vi "Relay.vi"(6 "Relay Mode":bool[](array[boolean]), 8 "error in":errorcluster, 9 "Relay Class":string="NI 6514\\NI 6514.lvclass", 10 "Line(s)":string="PXIe-6514/port4/line0:2", 11 "Base Path":path=path "C:/GitHub/OOP Template/HAL/Concrete") -> (0 "error out":errorcluster={"status"=TRUE, "code"=1446, "source"="Preserve Run-Time Class in MAL.lvlib:Relay.vi"})   [LabVIEW 2019, in "MAL.lvlib"]
uses:
  MAL.lvlib
  Hardware Abstraction/Harware Abstraction/DIO/DIO.lvclass
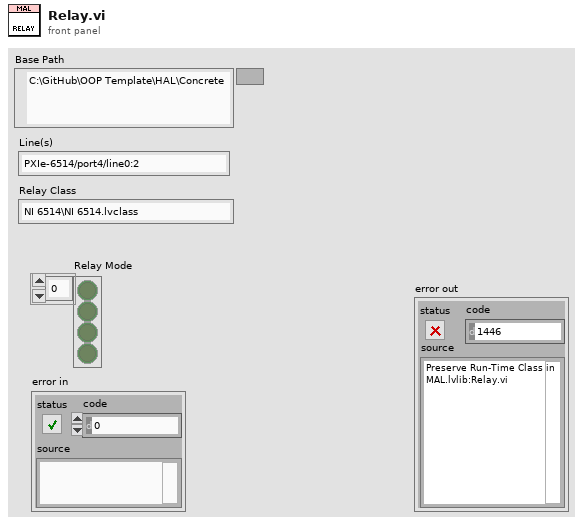
[diagram p1: front panel]
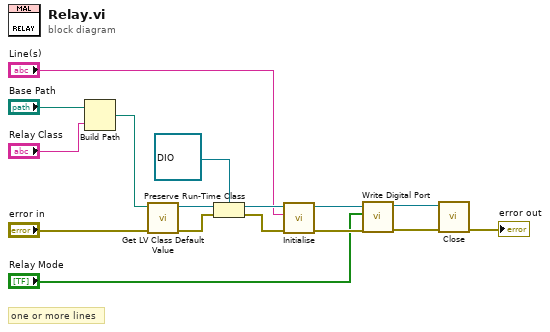
[diagram p0: block diagram]
diagram:
  # "one or more lines"
  n1 = Build Path(base path="Base Path", name or relative path="Relay Class") -> (appended path=w14:path)
  n2 = call <vilib>:"Get LV Class Default Value.vi"("error in (no error)"="error in", "class path"=w14) -> ("error out"=w12:errorcluster, "object"=w11:refnum<class>)  [unwired: 8 in]
  n3 = Preserve Run-Time Class(object in=w11, error in=w12, 2:refnum<class "DIO.lvclass"> refnum ("Hardware Abstration.lvlib:DIO.lvclass")) -> (object out=w10:refnum<class "DIO.lvclass">, error out=w8:errorcluster)
  n4 = call-dynamic "Initialise.vi"("error in (no error)"=w8, "Instrument Ref"="Line(s)", "Instrument in"=w10) -> ("error out"=w7:errorcluster, "Instrument out"=w6:refnum<class "DIO.lvclass">)  [unwired: 7 in]
  n5 = call-dynamic "Write Digital Port.vi"("error in (no error)"=w7, "Relay Mode"="Relay Mode", "DIO in"=w6) -> ("error out"=w3:errorcluster, "DIO out"=w4:refnum<class "DIO.lvclass">)  [unwired: 7 in]
  n6 = call-dynamic "Close.vi"("error in (no error)"=w3, "Instrument in"=w4) -> ("error out"=→"error out":errorcluster)  [unwired: 8 in, 1 out]
